vi "Reset Display.vi"(11 "Reset Button":bool) -> (1 "YScale Fit":dbl, 3 "XScale Fit":dbl)   [LabVIEW 2013]
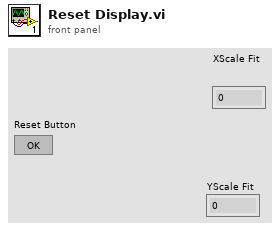
[diagram p1: front panel]
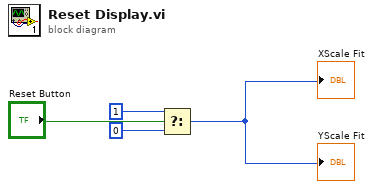
[diagram p0: block diagram]
diagram:
  n1 = Select(t=1, s="Reset Button", f=0) -> (s? t:f=→"XScale Fit" →"YScale Fit":i32)
